vi "~file record search.vi"() -> ()   [LabVIEW 2017]
panel:
  out ">=":bool
  out "!= True":bool
  out "i":i32
  out "Module found":i32
  in  "Module":i32
  in  "Modules":i32[](array[numeric])
  in  "Current Record":T1 {"Atten" format="%.3g"; "PS" format="%.3g"}
  in  "Existing Sequence":T2(array[cluster]) {"Atten" format="%.3g"; "PS" format="%.3g"}
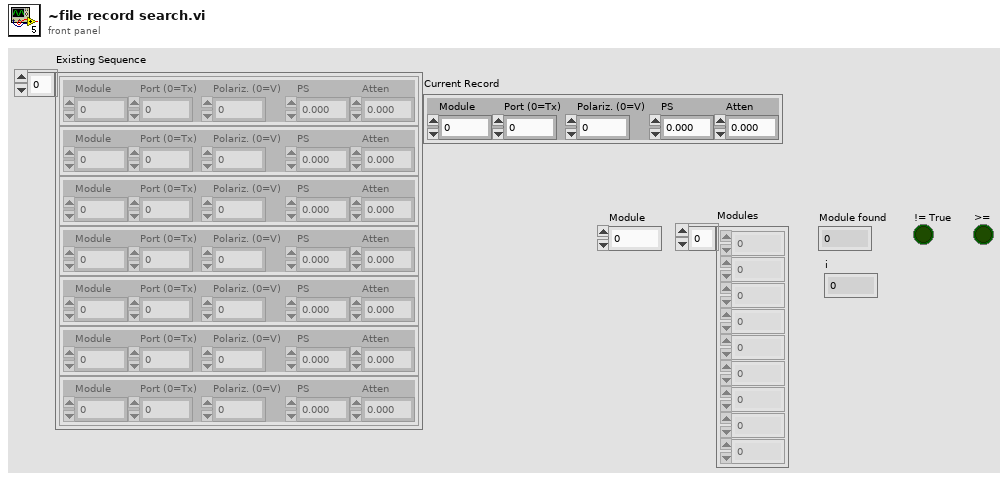
[diagram p1: front panel]
types:
  T1 = cluster{"Module":dbl, "Port (0=Tx)":dbl, "Polariz. (0=V)":dbl, "PS":dbl, "Atten":dbl}
  T2 = cluster{"Module":dbl, "Port (0=Tx)":dbl, "Polariz. (0=V)":dbl, "PS":dbl, "Atten":dbl}[]
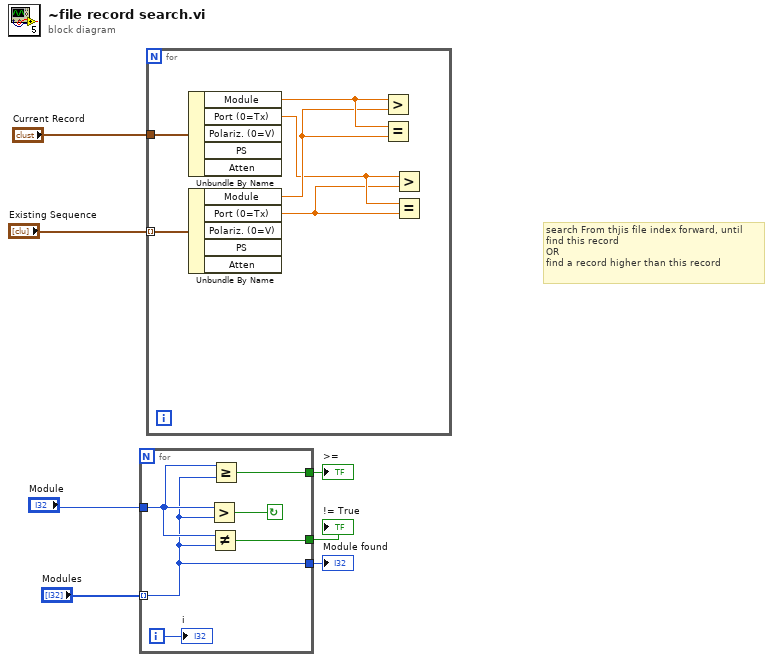
[diagram p0: block diagram]
diagram:
  # "search From thjis file index forward, until \nfind this record \nOR\nfind a record higher than this record"
  n1 = for {
    tunnel: "Modules" -> [w9] mode=indexing
    tunnel: "Module" -> [w10]
    tunnel: [w9] -> w3
    tunnel: [w11] -> w2
    tunnel: [w8] -> w1
    i -> [w12]
    stop <- w13 continue-if-true
    n2 = Greater?(x=w10, y=w9) -> (0:w13:bool)
    n3 = Not Equal?(x=w10, y=w9) -> (x != y?=w11:bool)
    n4 = Greater Or Equal?(x=w10, y=w9) -> (x >= y?=w8:bool)
    "i" <- w12
  }
  "Module found" <- w3
  "!= True" <- w2
  ">=" <- w1
  n5 = for {
    tunnel: "Existing Sequence" -> [w19] mode=indexing
    tunnel: "Current Record" -> [w18]
    n6 = Unbundle By Name(w18) -> ("Module"=w17:dbl, "Port (0=Tx)"=w15:dbl)  [unwired: 3 out]
    n7 = Unbundle By Name(w19) -> ("Module"=w16:dbl, "Port (0=Tx)"=w14:dbl)  [unwired: 3 out]
    n8 = Greater?(x=w17, y=w16) -> ()  [unwired: 1 out]
    n9 = Equal?(x=w17, y=w16) -> ()  [unwired: 1 out]
    n10 = Greater?(x=w15, y=w14) -> ()  [unwired: 1 out]
    n11 = Equal?(x=w15, y=w14) -> ()  [unwired: 1 out]
  }
